vi "Ctor.vi"(6 "Debug? (F)":bool, 8 "error in (no error)":errorcluster, 10 "Create Engine? (T)":bool=TRUE, 11 "TS License Type (Operator)":T1) -> (0 "error out":errorcluster, 3 "TSnax UI Manager out":refnum<class "TSnax UI Manager.lvclass">, 5 "Engine":refnum<class "Engine.lvclass">)   [LabVIEW 2020, in "TSnax UI.lvlib" / "TSnax UI Manager.lvclass"]
uses:
  TSnax UI Manager.lvclass
  TSnax/TS License Type.ctl
  TSnax/Engine/Engine.lvclass
  TSnax UI Manager.lvclass/TSnax UI Manager.ctl
  <vilib>/IlluminatedG/IG OOPanel/OOPanel/Manager/Manager.lvclass
  TSnax/TSnax.lvlib
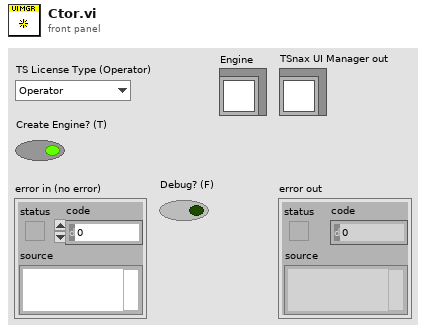
[diagram p1: front panel]
types:
  T1 = typedef "TSnax.lvlib/TS License Type.ctl" = enum16{"Operator", "CustomEditor", "SequenceEditor"}
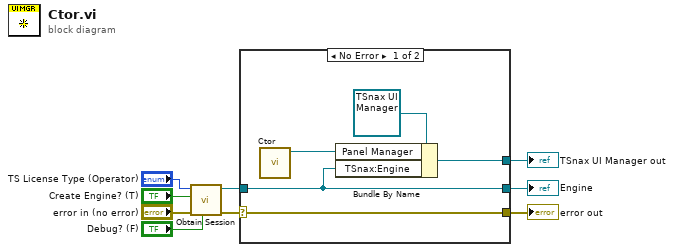
[diagram p0: block diagram]
diagram:
  n1 = call "Obtain Session.vi"("Debug Daemon (Dev Only)"="Debug? (F)", "error in (no error)"="error in (no error)", "Create if needed? (T)"="Create Engine? (T)", "TS License Type (Operator)"="TS License Type (Operator)") -> ("error out"=w4:errorcluster, "Engine out"=w3:refnum<class "Engine.lvclass">)  [unwired: 6 in]
  n2 = case shown="No Error" w4 {
    selector: w4 -> [w11 w15]
    tunnel: [w13 _] -> w9
    tunnel: w3 -> [w10 _]
    tunnel: [w11 w15] -> w2
    tunnel: [w10 _] -> w1
    frame No Error {
      n3 = call <vilib>:"Ctor.vi"() -> ("Manager out"=w12:refnum<class "Manager.lvclass">)  [unwired: 10 in, 1 out]
      n4 = Bundle By Name(cluster=refnum<class "TSnax UI Manager.lvclass"> refnum ("TSnax UI Manager in"), "Panel Manager"=w12, "TSnax:Engine"=w10) -> (w13:refnum<class "TSnax UI Manager.lvclass">)
    }
    frame Error {
    }
  }
  "error out" <- w2
  "TSnax UI Manager out" <- w9
  "Engine" <- w1
